vi "AVTCP-Sample Rate FGV.vi"(4 "Value in":dbl, 5 "Action":T1=enum."Write") -> (0 "Value out":dbl)   [LabVIEW 2020]
uses:
  AVTCP-FGV Action.ctl
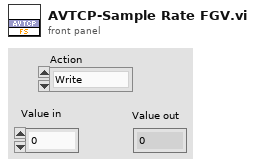
[diagram p1: front panel]
types:
  T1 = typedef "AVTCP-FGV Action.ctl" = enum16{"Init", "Write", "Read"}
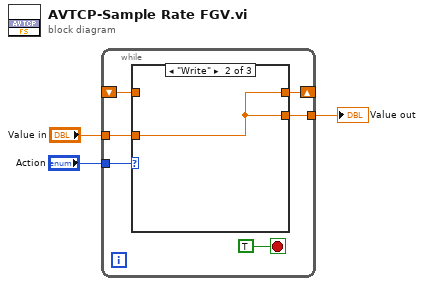
[diagram p0: block diagram]
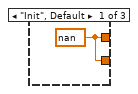
[diagram p2: hidden frame]
diagram:
  n1 = while {
    tunnel: "Action" -> [w9]
    tunnel: "Value in" -> [w7]
    shift-right: [w8] -> _
    shift-left: _ -> [w6]
    tunnel: [w5] -> w1
    stop <- TRUE stop-if-true
    n2 = case shown="\"Write\"" w9 {
      tunnel: [w10 w11 w12] -> w8
      tunnel: w7 -> [_ w11 _]
      tunnel: w6 -> [_ _ w12]
      tunnel: [w10 w11 w12] -> w5
      frame "Init", Default {
        w10 = nan
      }
      frame "Write" {
      }
      frame "Read" {
      }
    }
  }
  "Value out" <- w1
